vi "setLaserPower.vi"(8 "error in (no error)":errorcluster, 10 "power":dbl, 11 "Monochromator in":refnum<class "Monochromator.lvclass">) -> (0 "error out":errorcluster, 1 "ID":i32, 2 "results-JSON string":string, 3 "Monochromator out":refnum<class "Monochromator.lvclass">)   [LabVIEW 2023, in "Monochromator.lvclass"]
uses:
  Monochromator.lvclass
  7fe8abea-6ecd-46de-aa11-ce8637911b6a.vi
  35d46a5a-fd7c-4445-96f4-e877dae8f93b.vi
  <vilib>/JDP Science/JSONtext/Variant to JSON Text.vi
  <vilib>/JDP Science/JSONtext/Set Item.vi
  <vilib>/JDP Science/JSONtext/LVClass Serializer/JSONtext LVClass Serializer.lvclass
  Monochromator.lvclass/Monochromator.ctl
  GenericDevice/GenericDevice.lvclass
  <vilib>/IlluminatedG/lv-web-crypto/lv-json/JSON/JSON.lvlib
panel:
  # "Connector Pane"
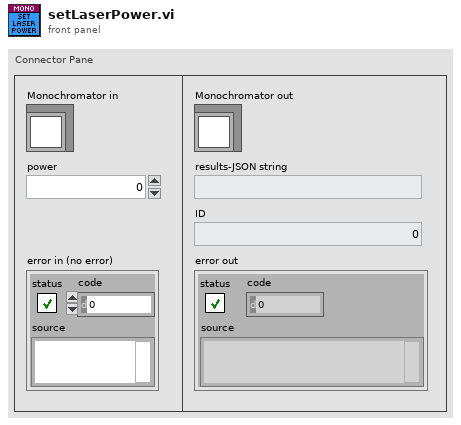
[diagram p1: front panel]
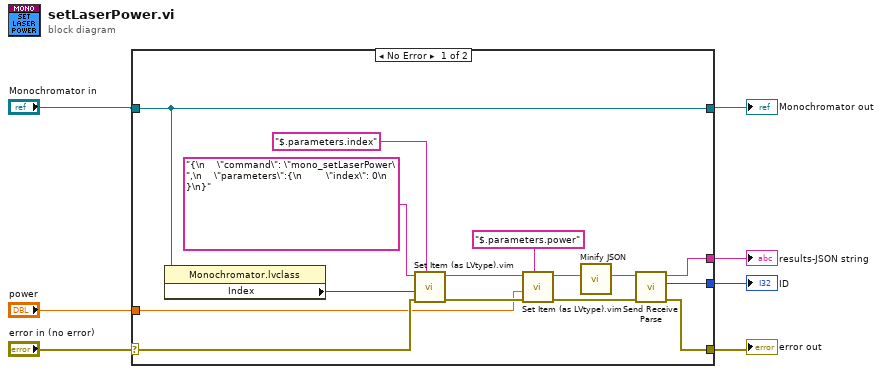
[diagram p0: block diagram]
diagram:
  n1 = case shown="No Error" "error in (no error)" {
    selector: "error in (no error)" -> [w18 w24]
    tunnel: [w15 w24] -> w4
    tunnel: [w20 w23] -> w6
    tunnel: "Monochromator in" -> [w20 w23]
    tunnel: [w17 _] -> w2
    tunnel: [w16 _] -> w3
    tunnel: "power" -> [w8 _]
    frame No Error {
      n2 = property class="Monochromator.lvclass"(reference=w20) -> ("Index"=w19:i32)  [unwired: 1 in, 2 out]
      n3 = call "Set Item (as LVtype).vim"("$Path or Item Name"="$.parameters.index", "error in (no error)"=w18, "Anything"=w19, "JSON"="{\n    \"command\": \"mono_setLaserPower\",\n    \"parameters\":{\n        \"index\": 0\n    }\n}") -> ("error out"=w12:errorcluster, "<JSON>"=w10:string)  [unwired: 4 in, 1 out]
      n4 = call "Set Item (as LVtype).vim"("$Path or Item Name"="$.parameters.power", "error in (no error)"=w12, "Anything"=w8, "JSON"=w10) -> ("error out"=w11:errorcluster, "<JSON>"=w9:string)  [unwired: 4 in, 1 out]
      n5 = call <vilib>:"Minify JSON.vi"("JSON String"=w9) -> ("Minified JSON"=w14:string)  [unwired: 10 in]
      n6 = call "Send Receive Parse.vi"("error in"=w11, "<JSON>"=w14) -> ("error out"=w15:errorcluster, "ID"=w16:i32, "results-JSON string"=w17:string)  [unwired: 7 in]
    }
    frame Error {
    }
  }
  "error out" <- w4
  "Monochromator out" <- w6
  "ID" <- w3
  "results-JSON string" <- w2
